vi "Lab Panel V5.27.vi"() -> ()   [LabVIEW 2013] (continued)
              w199 = T12 {"T1 Live"=20.0, "T1 Neut"=20.0, "T2 Live"=20.0, "T2 Neut"=20.0, "ID"=6.0, "ER"=10.0} ("LAB01 TEMP")
              n184 = local write "LAB deg C"(w199) -> ()
              n185 = global write "Global display 4.vi" "LAB deg C"(w199) -> ()
              n186 = local write "OFF amps"(1.5) -> ()
              n187 = local write "ON amps"(20.0) -> ()
              n188 = local write "VOLTS"(250.0) -> ()
              n189 = local write "PF"(0.5) -> ()
            }
            frame #1 {
              n190 = for {
                N: 3 -> [_]
                w245 = TRUE
                n191 = local read "Simulate"() -> (w207:bool)
                n192 = local write "Temp read loop"(0) -> ()
                n193 = case shown="True" w207 {
                  frame False {
                  }
                  frame True {
                    w247 = 20
                    n194 = local write "Ambient Volts"(2.92) -> ()
                    n195 = global write "Global display 3.vi" "Ref deg C"(w247) -> ()
                    n196 = local write "Ref deg C"(w247) -> ()
                  }
                }
                n197 = call "sub vi - GET ALL TEMP v7.vi"("LA01-EN"=w245, "simulate"=w207, "LA02-EN"=w245, "LA03-EN"=w245, "LA04-EN"=w245, "LA05-EN"=w245, "Gen Cal Value"=1) -> ("ID"=w206:T24, "LA01 TEMP"=w243:T25, "LA02 TEMP"=w236:T25, "LA03 TEMP"=w229:T25, "LA04 TEMP"=w222:T25, "LA05 TEMP"=w215:T25)  [unwired: 1 in, 2 out]
                n198 = local write "LAB05 TEMP"(w215) -> ()
                n199 = local write "LAB04 TEMP"(w222) -> ()
                n200 = Unbundle(w229) -> ("T1"=w226:dbl, "T2"=w225:dbl, "T3"=w224:dbl, "T4"=w223:dbl)  [unwired: 2 out]
                n201 = Unbundle(w243) -> ("T1"=w241:dbl, "T2"=w240:dbl, "T3"=w239:dbl, "T4"=w238:dbl)  [unwired: 2 out]
                n202 = Unbundle(w236) -> ("T1"=w233:dbl, "T2"=w232:dbl, "T3"=w231:dbl, "T4"=w230:dbl)  [unwired: 2 out]
                n203 = Unbundle(w222) -> ("T1"=w220:dbl, "T2"=w219:dbl, "T3"=w218:dbl, "T4"=w217:dbl)  [unwired: 2 out]
                n204 = Unbundle(w215) -> ("T1"=w213:dbl, "T2"=w212:dbl, "T3"=w211:dbl, "T4"=w210:dbl)  [unwired: 2 out]
                n205 = local write "LAB01 TEMP"(w243) -> ()
                n206 = local write "LAB02 TEMP"(w236) -> ()
                n207 = local write "LAB03 TEMP"(w229) -> ()
                n208 = Unbundle(w206) -> ("id1"=→"LAB01-TP":bool, "id2"=→"LAB02-TP":bool, "id3"=→"LAB03-TP":bool, "id4"=→"LAB04-TP":bool, "id5"=→"LAB05-TP":bool)
                n209 = local read "TEMP LA05"() -> (w214:T9)
                n210 = local read "TEMP LA04"() -> (w221:T9)
                n211 = local read "TEMP LA02"() -> (w235:T9)
                n212 = local read "TEMP LA03"() -> (w228:T9)
                n213 = local read "TEMP LA01"() -> (w242:T9)
                n214 = Bundle(cluster=w228, "TL-1"=w226, "TN-1"=w225, "TL-2"=w224, "TN-2"=w223) -> (w227:T9)  [unwired: 4 in]
                n215 = Bundle(cluster=w242, "TL-1"=w241, "TN-1"=w240, "TL-2"=w239, "TN-2"=w238) -> (w237:T9)  [unwired: 4 in]
                n216 = Bundle(cluster=w235, "TL-1"=w233, "TN-1"=w232, "TL-2"=w231, "TN-2"=w230) -> (w234:T9)  [unwired: 4 in]
                n217 = Bundle(cluster=w221, "TL-1"=w220, "TN-1"=w219, "TL-2"=w218, "TN-2"=w217) -> (w216:T9)  [unwired: 4 in]
                n218 = Bundle(cluster=w214, "TL-1"=w213, "TN-1"=w212, "TL-2"=w211, "TN-2"=w210) -> (w209:T9)  [unwired: 4 in]
                n219 = local write "TEMP LA03"(w227) -> ()
                n220 = local write "TEMP LA01"(w237) -> ()
                n221 = local write "TEMP LA02"(w234) -> ()
                n222 = local write "TEMP LA05"(w209) -> ()
                n223 = local write "TEMP LA04"(w216) -> ()
              }
            }
            frame #2 {
              w256 = 0
              n224 = local read "LAB01 TEMP"() -> (w258:T12)
              n225 = local read "SIG LAB01-2"() -> (w253:T2)
              n226 = Unbundle By Name(w258) -> ("T1 Live"=w251:dbl, "T1 Neut"=w250:dbl, "T2 Live"=w249:dbl, "T2 Neut"=w248:dbl)  [unwired: 2 out]
              n227 = local read "SIG LAB01-1"() -> (w255:T2)
              n228 = local read "TEMP LA01"() -> (w259:T9)
              n229 = Bundle By Name(cluster=w259, "TL-1"=w251, "TN-1"=w250, "TL-2"=w249, "TN-2"=w248, "TL -1COUNT"=w256, "TN-1 COUNT"=w256, "TL-2 COUNT"=w256, "TN-2 COUNT"=w256) -> (w257:T9)
              n230 = Bundle(cluster=w255, "Tmp Live"=w251, "Tmp Neut"=w250) -> (w254:T2)  [unwired: 3 in]
              n231 = Bundle(cluster=w253, "Tmp Live"=w249, "Tmp Neut"=w248) -> (w252:T2)  [unwired: 3 in]
              n232 = local write "SIG LAB01-2"(w252) -> ()
              n233 = local write "SIG LAB01-1"(w254) -> ()
              n234 = local write "TEMP LA01"(w257) -> ()
            }
            frame #3 {
              w268 = 0
              n235 = local read "LAB02 TEMP"() -> (w270:T12)
              n236 = Unbundle By Name(w270) -> ("T1 Live"=w263:dbl, "T1 Neut"=w262:dbl, "T2 Live"=w261:dbl, "T2 Neut"=w260:dbl)  [unwired: 2 out]
              n237 = local read "SIG LAB02-1"() -> (w267:T2)
              n238 = local read "SIG LAB02-2"() -> (w266:T2)
              n239 = local read "TEMP LA02"() -> (w271:T9)
              n240 = Bundle By Name(cluster=w271, "TL-1"=w263, "TN-1"=w262, "TL-2"=w261, "TN-2"=w260, "TL -1COUNT"=w268, "TN-1 COUNT"=w268, "TL-2 COUNT"=w268, "TN-2 COUNT"=w268) -> (w269:T9)
              n241 = Bundle(cluster=w266, "Tmp Live"=w261, "Tmp Neut"=w260) -> (w264:T2)  [unwired: 3 in]
              n242 = Bundle(cluster=w267, "Tmp Live"=w263, "Tmp Neut"=w262) -> (w265:T2)  [unwired: 3 in]
              n243 = local write "TEMP LA02"(w269) -> ()
              n244 = local write "SIG LAB02-1"(w265) -> ()
              n245 = local write "SIG LAB02-2"(w264) -> ()
            }
            frame #4 {
              w280 = 0
              n246 = local read "LAB03 TEMP"() -> (w282:T12)
              n247 = Unbundle By Name(w282) -> ("T1 Live"=w275:dbl, "T1 Neut"=w274:dbl, "T2 Live"=w273:dbl, "T2 Neut"=w272:dbl)  [unwired: 2 out]
              n248 = local read "SIG LAB03-1"() -> (w279:T2)
              n249 = local read "SIG LAB03-2"() -> (w278:T2)
              n250 = local read "TEMP LA03"() -> (w283:T9)
              n251 = Bundle By Name(cluster=w283, "TL-1"=w275, "TN-1"=w274, "TL-2"=w273, "TN-2"=w272, "TL -1COUNT"=w280, "TN-1 COUNT"=w280, "TL-2 COUNT"=w280, "TN-2 COUNT"=w280) -> (w281:T9)
              n252 = Bundle(cluster=w278, "Tmp Live"=w273, "Tmp Neut"=w272) -> (w276:T2)  [unwired: 3 in]
              n253 = Bundle(cluster=w279, "Tmp Live"=w275, "Tmp Neut"=w274) -> (w277:T2)  [unwired: 3 in]
              n254 = local write "TEMP LA03"(w281) -> ()
              n255 = local write "SIG LAB03-2"(w276) -> ()
              n256 = local write "SIG LAB03-1"(w277) -> ()
            }
            frame #5 {
              w292 = 0
              n257 = local read "LAB04 TEMP"() -> (w294:T12)
              n258 = Unbundle By Name(w294) -> ("T1 Live"=w287:dbl, "T1 Neut"=w286:dbl, "T2 Live"=w285:dbl, "T2 Neut"=w284:dbl)  [unwired: 2 out]
              n259 = local read "SIG LAB04-2"() -> (w290:T2)
              n260 = local read "SIG LAB04-1"() -> (w291:T2)
              n261 = local read "TEMP LA04"() -> (w295:T9)
              n262 = Bundle By Name(cluster=w295, "TL-1"=w287, "TN-1"=w286, "TL-2"=w285, "TN-2"=w284, "TL -1COUNT"=w292, "TN-1 COUNT"=w292, "TL-2 COUNT"=w292, "TN-2 COUNT"=w292) -> (w293:T9)
              n263 = Bundle(cluster=w290, "Tmp Live"=w285, "Tmp Neut"=w284) -> (w288:T2)  [unwired: 3 in]
              n264 = Bundle(cluster=w291, "Tmp Live"=w287, "Tmp Neut"=w286) -> (w289:T2)  [unwired: 3 in]
              n265 = local write "SIG LAB04-2"(w288) -> ()
              n266 = local write "TEMP LA04"(w293) -> ()
              n267 = local write "SIG LAB04-1"(w289) -> ()
            }
            frame #6 {
              w304 = 0
              n268 = local read "LAB05 TEMP"() -> (w306:T12)
              n269 = Unbundle By Name(w306) -> ("T1 Live"=w299:dbl, "T1 Neut"=w298:dbl, "T2 Live"=w297:dbl, "T2 Neut"=w296:dbl)  [unwired: 2 out]
              n270 = local read "SIG LAB05-2"() -> (w302:T2)
              n271 = local read "SIG LAB05-1"() -> (w303:T2)
              n272 = local read "TEMP LA05"() -> (w307:T9)
              n273 = Bundle By Name(cluster=w307, "TL-1"=w299, "TN-1"=w298, "TL-2"=w297, "TN-2"=w296, "TL -1COUNT"=w304, "TN-1 COUNT"=w304, "TL-2 COUNT"=w304, "TN-2 COUNT"=w304) -> (w305:T9)
              n274 = Bundle(cluster=w302, "Tmp Live"=w297, "Tmp Neut"=w296) -> (w300:T2)  [unwired: 3 in]
              n275 = Bundle(cluster=w303, "Tmp Live"=w299, "Tmp Neut"=w298) -> (w301:T2)  [unwired: 3 in]
              n276 = local write "SIG LAB05-2"(w300) -> ()
              n277 = local write "SIG LAB05-1"(w301) -> ()
              n278 = local write "TEMP LA05"(w305) -> ()
            }
          }
        }
        frame #11 {
          # "create analog task"
          n279 = local read "Simulate"() -> (w308:bool)
          n280 = case shown="False" w308 {
            frame False {
              n281 = local read "SAMPLES"() -> (w310:dbl)
              n282 = local read "RATE (Hz)"() -> (w311:dbl)
              n283 = local read "AI Task0"() -> (w314:dbl)
              n284 = local read "AI Task2"() -> (w312:dbl)
              n285 = local read "AI Task1"() -> (w313:dbl)
              n286 = call "sub vi - AI USB4704 (3)  Create Task v3.vi"("Task In 0"=w314, "Task In 1"=w313, "Task In 2"=w312, "Rate Hz"=w311, "Samples"=w310) -> ("TASK USB 0"=→"AI Task0":i32, "TASK USB 1"=→"AI Task1":i32, "TASK USB 2"=→"AI Task2":i32, "AI Task Er"=→"AI Task":bool)  [unwired: 6 in, 1 out]
            }
            frame True {
            }
          }
        }
        frame #12 {
          # "enable front panel, all settings done"
          n287 = property on="Tab Control 2" class="TabCtl (strict)"("DisabledEnum"=T16."Enabled" ("Disabled")) -> ()  [unwired: 2 in, 2 out]
          n288 = property on="Tab Control 2" class="TabCtl (strict)"("Value"=0) -> ()  [unwired: 2 in, 2 out]
        }
        frame #13 {
          n289 = property on="Tab Control 2" class="TabCtl (strict)"("Value"=0) -> ()  [unwired: 2 in, 2 out]
        }
      }
    }
    frame #2 {
      w321 = 250.0
      # "frames that only action on certain cycles, 13, 14, 15, 16, 19, 21"
      n290 = node-c288(w321) -> (w323:T18)  [unwired: 3 in]
      n291 = timed-loop {
        timing: w323 -> [_]
        timing-out: [_] -> w322
        tunnel: w321 -> [w324]
        i -> [w350]
        stop <- w325 stop-if-true
        n292 = node-c288() -> ()  [unwired: 1 in, 1 out]
        n293 = local read "Resets Done"() -> (w329:dbl)
        n294 = local read "SELECT LAB05-2"() -> (w330:T3)
        n295 = local read "SELECT LAB05-1"() -> (w331:T3)
        n296 = local read "SELECT LAB04-2"() -> (w332:T3)
        n297 = local read "SELECT LAB03-1"() -> (w335:T3)
        n298 = local read "SELECT LAB02-2"() -> (w336:T3)
        n299 = local read "SELECT LAB01-1"() -> (w339:T3)
        n300 = local read "SELECT LAB03-2"() -> (w334:T3)
        n301 = local read "SELECT LAB01-2"() -> (w338:T3)
        n302 = local read "SELECT LAB04-1"() -> (w333:T3)
        n303 = Greater?(x=w329, y=50) -> (0:w326:bool)
        n304 = local read "SELECT LAB02-1"() -> (w337:T3)
        n305 = local read "run lab03-2"() -> (w344:bool)
        n306 = local read "run lab04-1"() -> (w343:bool)
        n307 = local read "run lab05-1"() -> (w341:bool)
        n308 = local read "run lab04-2"() -> (w342:bool)
        n309 = local read "run lab05-2"() -> (w340:bool)
        n310 = local read "run lab03-1"() -> (w345:bool)
        n311 = local read "run lab02-2"() -> (w346:bool)
        n312 = local read "run lab02-1"() -> (w347:bool)
        n313 = local read "run lab01-1"() -> (w349:bool)
        n314 = local read "run lab01-2"() -> (w348:bool)
        n315 = Or(x=w326, y="stop") -> (x .or. y?=w325:bool)
        n316 = global write "Global display 1.vi" "stop disp"(w325) -> ()
        n317 = stacked-sequence {
          seq-local: [_ _ w429 _ _ _ _ _ _ _ _ _ _ _ _ _ _ _ _ _ _ _ _ _ _] -> [_ _ _ _ _ _ w2530 _ _ _ _ _ _ _ _ _ _ _ _ _ _ _ _ _ _]
          seq-local: [_ _ w428 _ _ _ _ _ _ _ _ _ _ _ _ _ _ _ _ _ _ _ _ _ _] -> [_ _ _ _ _ _ w2529 _ _ _ _ _ _ _ _ _ _ _ _ _ _ _ _ _ _]
          seq-local: [_ _ w415 _ _ _ _ _ _ _ _ _ _ _ _ _ _ _ _ _ _ _ _ _ _] -> [_ _ _ _ _ _ w2528 _ _ _ _ _ _ _ _ _ _ _ _ _ _ _ _ _ _]
          seq-local: [_ _ w414 _ _ _ _ _ _ _ _ _ _ _ _ _ _ _ _ _ _ _ _ _ _] -> [_ _ _ _ _ _ w2527 _ _ _ _ _ _ _ _ _ _ _ _ _ _ _ _ _ _]
          seq-local: [_ _ w413 _ _ _ _ _ _ _ _ _ _ _ _ _ _ _ _ _ _ _ _ _ _] -> [_ _ _ _ _ _ w2526 _ _ _ _ _ _ _ _ _ _ _ _ _ _ _ _ _ _]
          seq-local: [_ _ w412 _ _ _ _ _ _ _ _ _ _ _ _ _ _ _ _ _ _ _ _ _ _] -> [_ _ _ _ _ _ w2525 _ _ _ _ _ _ _ _ _ _ _ _ _ _ _ _ _ _]
          seq-local: [_ _ w411 _ _ _ _ _ _ _ _ _ _ _ _ _ _ _ _ _ _ _ _ _ _] -> [_ _ _ _ _ _ w2524 _ _ _ _ _ _ _ _ _ _ _ _ _ _ _ _ _ _]
          seq-local: [_ _ w410 _ _ _ _ _ _ _ _ _ _ _ _ _ _ _ _ _ _ _ _ _ _] -> [_ _ _ _ _ _ w2523 _ _ _ _ _ _ _ _ _ _ _ _ _ _ _ _ _ _]
          seq-local: [_ _ w409 _ _ _ _ _ _ _ _ _ _ _ _ _ _ _ _ _ _ _ _ _ _] -> [_ _ _ _ _ _ w2522 _ _ _ _ _ _ _ _ _ _ _ _ _ _ _ _ _ _]
          seq-local: [_ _ w408 _ _ _ _ _ _ _ _ _ _ _ _ _ _ _ _ _ _ _ _ _ _] -> [_ _ _ _ _ _ w2521 _ _ _ _ _ _ _ _ _ _ _ _ _ _ _ _ _ _]
          seq-local: [_ _ _ _ _ _ _ _ _ _ _ _ w3667 _ _ _ _ _ _ _ _ _ _ _ _] -> [_ _ _ _ _ _ _ _ _ _ _ _ _ w3725 _ _ _ _ _ _ _ _ _ _ _]
          tunnel: w349 -> [_ _ _ w445 w693 w2120 w2550 w2866 w3353 _ _ _ _ _ w4009 _ w4966 _ _ w5254 w5558 w5739 _ _ _]
          tunnel: w348 -> [_ _ _ w444 w691 w2119 w2549 w2867 w3352 _ _ _ _ _ w4008 _ w4964 _ _ w5253 w5557 w5737 _ _ _]
          tunnel: w347 -> [_ _ _ w443 w689 w2118 w2548 w2865 w3351 _ _ _ _ _ w4007 _ w4962 _ _ w5252 w5556 w5736 _ _ _]
          tunnel: w346 -> [_ _ _ w442 w687 w2117 w2547 w2864 w3350 _ _ _ _ _ w4006 _ w4960 _ _ w5251 w5555 w5735 _ _ _]
          tunnel: w345 -> [_ _ _ w441 w685 w2116 w2546 w2863 w3349 _ _ _ _ _ w4005 _ w4958 _ _ w5250 w5554 w5734 _ _ _]
          tunnel: w344 -> [_ _ _ w440 w683 w2115 w2545 w2862 w3348 _ _ _ _ _ w4004 _ w4956 _ _ w5249 w5553 w5733 _ _ _]
          tunnel: w343 -> [_ _ _ w439 w681 w2114 w2544 w2861 w3347 _ _ _ _ _ w4003 _ w4954 _ _ w5248 w5552 w5732 _ _ _]
          tunnel: w342 -> [_ _ _ w438 w679 w2113 w2543 w2860 w3346 _ _ _ _ _ w4002 _ w4952 _ _ w5247 w5551 w5731 _ _ _]
          tunnel: w341 -> [_ _ _ w437 w677 w2112 w2542 w2859 w3345 _ _ _ _ _ w4001 _ w4950 _ _ w5246 w5550 w5730 _ _ _]
          tunnel: w340 -> [_ _ _ w436 w675 w2111 w2541 w2858 w3344 _ _ _ _ _ w4000 _ w4948 _ _ w5245 w5549 w5729 _ _ _]
          tunnel: w339 -> [_ _ _ _ w692 w2110 w2540 _ _ _ _ _ _ _ _ _ w4968 _ _ _ _ _ w6195 _ _]
          tunnel: w338 -> [_ _ _ _ w690 w2109 w2539 _ _ _ _ _ _ _ _ _ w4963 _ _ _ _ _ w6194 _ _]
          tunnel: w337 -> [_ _ _ _ w688 w2108 w2538 _ _ _ _ _ _ _ _ _ w4961 _ _ _ _ _ w6193 _ _]
          tunnel: w336 -> [_ _ _ _ w686 w2107 w2537 _ _ _ _ _ _ _ _ _ w4959 _ _ _ _ _ w6192 _ _]
          tunnel: w335 -> [_ _ _ _ w684 w2106 w2536 _ _ _ _ _ _ _ _ _ w4957 _ _ _ _ _ w6191 _ _]
          tunnel: w334 -> [_ _ _ _ w682 w2105 w2535 _ _ _ _ _ _ _ _ _ w4955 _ _ _ _ _ w6190 _ _]
          tunnel: w333 -> [_ _ _ _ w680 w2104 w2534 _ _ _ _ _ _ _ _ _ w4953 _ _ _ _ _ w6189 _ _]
          tunnel: w332 -> [_ _ _ _ w678 w2103 w2533 _ _ _ _ _ _ _ _ _ w4951 _ _ _ _ _ w6188 _ _]
          tunnel: w331 -> [_ _ _ _ w676 w2102 w2532 _ _ _ _ _ _ _ _ _ w4949 _ _ _ _ _ w6187 _ _]
          tunnel: w330 -> [_ _ _ _ w674 w2101 w2531 _ _ _ _ _ _ _ _ _ w4947 _ _ _ _ _ w6186 _ _]
          tunnel: w326 -> [_ _ _ _ _ _ _ _ _ _ _ _ _ _ _ _ _ _ _ _ _ _ _ _ w6298]
          tunnel: w325 -> [_ _ _ _ _ _ _ _ _ _ _ _ _ _ _ _ _ _ _ _ _ _ _ _ w6297]
          tunnel: w324 -> [_ w365 _ _ _ _ _ _ _ _ _ _ _ _ _ _ _ _ _ _ _ _ _ _ _]
          frame #0 {
            n318 = local read "AI Task"() -> (w353:bool)
            n319 = global write "Global 1.vi" "RATE(Hz)"("RATE (Hz)") -> ()
            n320 = case shown="True" w353 {
              frame False {
              }
              frame True {
                n321 = local read "AI Task2"() -> (w361:dbl)
                n322 = local read "AI Task1"() -> (w362:dbl)
                n323 = local read "AI Task0"() -> (w363:dbl)
                n324 = call "sub vi - AI USB4704 (3) v73.vi"("Task0"=w363, "Task1"=w362, "Task2"=w361, "SAMPLES"="SAMPLES 2") -> ("data 0"=→"AI data 0" →"AI Data 0":waveform(dbl)[], "data 1"=→"AI data 1" →"AI Data 1":waveform(dbl)[], "data 2"=→"AI data 2" →"AI Data 2":waveform(dbl)[], "loop time"=→"AI loop time":dbl, "error array"=→"AI Error":errorcluster[])  [unwired: 7 in]
              }
            }
          }
          frame #1 {
            w372 = FALSE
            # "set up cycle control"
            n325 = local read "jig cycle"() -> (w376:dbl)
            n326 = local read "Amps Fail level"() -> (w370:dbl)
            n327 = local read "Simulate"() -> (w367:bool)
            n328 = Divide(x=w365, y=1000.0) -> (x/y=w364:dbl)
            n329 = Divide(x="JIG ON TIME (S)", y=w364) -> (x/y=→"on loops":dbl)
            n330 = Divide(x="JIG OFF TIME (S)", y=w364) -> (x/y=→"off loops":dbl)
            n331 = Increment(x=w376) -> (x+1=w375:dbl)
            n332 = local write "Simulate IND"(w367) -> ()
            n333 = global write "Global display 3.vi" "Amps Fail"(w370) -> ()
            n334 = local write "TEMP"(w372) -> ()
            n335 = local write "AI"(w372) -> ()
            n336 = local read "Network Directory"() -> (w369:path)
            n337 = local write "jig cycle"(w375) -> ()
            n338 = call "sub vi - check network dir v2.vi"("PATH"=w369) -> ("error"=w368:bool)  [unwired: 10 in]
            n339 = local write "network error"(w368) -> ()
            n340 = global write "Global display 3.vi" "network drive"(w368) -> ()
            n341 = event shown="[1] \"ADMIN\": Value Change" {
              selector: _ -> [_ _]
              dyn-events: _ -> [_ _]
              timeout: 10 -> [_ _]
              event Timeout {
                n342 = event-data() -> ()  [unwired: 1 in, 3 out]
              }
              event "ADMIN": Value Change {
                n343 = event-data() -> ()  [unwired: 1 in, 6 out]
                n344 = stacked-sequence {
                  seq-local: [_ w380 _] -> [_ _ w381]
                  frame #0 {
                    n345 = global write "Global 1.vi" "password"("9949") -> ()
                  }
                  frame #1 {
                    n346 = call "sub vi - password 1.vi"() -> ("RESULT"=w380:bool)  [unwired: 11 in]
                  }
                  frame #2 {
                    w383 = FALSE
                    n347 = property on="Tab Control 2" class="TabCtl (strict)"() -> ("Pages"=w387:refnum<vi>[])  [unwired: 2 in, 2 out]
                    n348 = Select(t=TRUE, s=w381, f=w383) -> (s? t:f=w382:bool)
                    n349 = Index Array(array=w387, index=8) -> (element=w385:refnum<vi>)
                    n350 = property class="Page"(reference=w385, "PageVis"=w382) -> ()  [unwired: 1 in, 2 out]
                    n351 = local write "ADMIN"(w383) -> ()
                  }
                }
              }
            }
          }
          frame #2 {
            w425 = 60.0
            # "convert temperature rise minutes to cycles"
            n352 = local read "SET LAB05-2"() -> (w389:T5)
            n353 = local read "SET LAB05-1"() -> (w391:T5)
            n354 = local read "SET LAB04-2"() -> (w393:T5)
            n355 = local read "SET LAB01-1"() -> (w407:T5)
            n356 = local read "SET LAB01-2"() -> (w405:T5)
            n357 = local read "SET LAB02-2"() -> (w401:T5)
            n358 = local read "SET LAB04-1"() -> (w395:T5)
            n359 = local read "SET LAB03-1"() -> (w399:T5)
            n360 = local read "SET LAB03-2"() -> (w397:T5)
            n361 = local read "SET LAB02-1"() -> (w403:T5)
            n362 = local read "JIG OFF TIME (S)"() -> (w430:dbl)
            n363 = local read "JIG ON TIME (S)"() -> (w431:dbl)
            n364 = Unbundle(w389) -> ("T-RISE mins"=w388:dbl)  [unwired: 4 out]
            n365 = Unbundle(w391) -> ("T-RISE mins"=w390:dbl)  [unwired: 4 out]
            n366 = Unbundle(w407) -> ("T-RISE mins"=w406:dbl)  [unwired: 4 out]
            n367 = Unbundle(w393) -> ("T-RISE mins"=w392:dbl)  [unwired: 4 out]
            n368 = Unbundle(w405) -> ("T-RISE mins"=w404:dbl)  [unwired: 4 out]
            n369 = Unbundle(w403) -> ("T-RISE mins"=w402:dbl)  [unwired: 4 out]
            n370 = Unbundle(w395) -> ("T-RISE mins"=w394:dbl)  [unwired: 4 out]
            n371 = Unbundle(w401) -> ("T-RISE mins"=w400:dbl)  [unwired: 4 out]
            n372 = Unbundle(w397) -> ("T-RISE mins"=w396:dbl)  [unwired: 4 out]
            n373 = Unbundle(w399) -> ("T-RISE mins"=w398:dbl)  [unwired: 4 out]
            n374 = Add(x=w431, y=w430) -> (x+y=w424:dbl)
            n375 = Multiply(x=w425, y=w396) -> (x*y=w420:dbl)
            n376 = Multiply(x=w425, y=w394) -> (x*y=w419:dbl)
            n377 = Multiply(x=w425, y=w392) -> (x*y=w418:dbl)
            n378 = Multiply(x=w425, y=w390) -> (x*y=w417:dbl)
            n379 = Multiply(x=w425, y=w388) -> (x*y=w416:dbl)
            n380 = Multiply(x=w425, y=w404) -> (x*y=w426:dbl)
            n381 = Multiply(x=w425, y=w398) -> (x*y=w421:dbl)
            n382 = Multiply(x=w425, y=w406) -> (x*y=w427:dbl)
            n383 = Multiply(x=w425, y=w402) -> (x*y=w423:dbl)
            n384 = Multiply(x=w425, y=w400) -> (x*y=w422:dbl)
            n385 = Divide(x=w417, y=w424) -> (x/y=w409:dbl)
            n386 = Divide(x=w418, y=w424) -> (x/y=w410:dbl)
            n387 = Divide(x=w419, y=w424) -> (x/y=w411:dbl)
            n388 = Divide(x=w416, y=w424) -> (x/y=w408:dbl)
            n389 = Divide(x=w421, y=w424) -> (x/y=w413:dbl)
            n390 = Divide(x=w427, y=w424) -> (x/y=w429:dbl)
            n391 = Divide(x=w426, y=w424) -> (x/y=w428:dbl)
            n392 = Divide(x=w423, y=w424) -> (x/y=w415:dbl)
            n393 = Divide(x=w422, y=w424) -> (x/y=w414:dbl)
            n394 = Divide(x=w420, y=w424) -> (x/y=w412:dbl)
          }
          frame #3 {
            # "control cycle loops"
            n395 = local read "JIG OFF TIME (S)"() -> (w434:dbl)
            n396 = local read "JIG ON TIME (S)"() -> (w433:dbl)
            n397 = local read "jig cycle"() -> (w447:dbl)
            n398 = local read "on loops"() -> (w449:dbl)
            n399 = local read "off loops"() -> (w448:dbl)
            n400 = Add(x=w434, y=w433) -> (x+y=w432:dbl)
            n401 = Add(x=w449, y=w448) -> (x+y=w435:dbl)
            n402 = Greater Or Equal?(x=w447, y=w435) -> (x >= y?=w446:bool)
            n403 = case shown="True" w446 {
              tunnel: w445 -> [_ w483]
              tunnel: w444 -> [_ w482]
              tunnel: w443 -> [_ w481]
              tunnel: w442 -> [_ w480]
              tunnel: w441 -> [_ w479]
              tunnel: w440 -> [_ w478]
              tunnel: w439 -> [_ w477]
              tunnel: w438 -> [_ w476]
              tunnel: w437 -> [_ w475]
              tunnel: w436 -> [_ w474]
              tunnel: w432 -> [_ w473]
              frame False {
              }
              frame True {
                # "increment cycle value and convert cycles to minutes for temp rise"
                n404 = stacked-sequence {
                  frame #0 {
                    n405 = local read "Temp read loop"() -> (w486:dbl)
                    n406 = Increment(x=w486) -> (x+1=w485:dbl)
                    n407 = local write "Temp read loop"(w485) -> ()
                  }
                  frame #1 {
                    n408 = local read "Temp read loop"() -> (w487:dbl)
                    n409 = Greater?(x=w487, y=20) -> (0:w489:bool)
                    n410 = case shown="True" w489 {
                      frame False {
                      }
                      frame True {
                        n411 = local write "Temp read loop"(1) -> ()
                      }
                    }
                  }
                }
                n412 = local read "JIG RELAY CYCLES"() -> (w472:T8)
                n413 = local read "Temp read loop"() -> (→"Tp Up":dbl)
                n414 = Unbundle By Name(w472) -> ("LAB01-1"=w470:dbl, "LAB01-2"=w468:dbl, "LAB02-1"=w466:dbl, "LAB02-2"=w464:dbl, "LAB03-1"=w462:dbl, "LAB03-2"=w460:dbl, "LAB04-1"=w458:dbl, "LAB04-2"=w456:dbl, "LAB05-1"=w454:dbl, "LAB05-2"=w452:dbl)
                n415 = stacked-sequence {
                  tunnel: w483 -> [w501 _ _ _ _ _ _ _ _ _]
                  tunnel: w482 -> [_ w518 _ _ _ _ _ _ _ _]
                  tunnel: w481 -> [_ _ w535 _ _ _ _ _ _ _]
                  tunnel: w480 -> [_ _ _ w552 _ _ _ _ _ _]
                  tunnel: w479 -> [_ _ _ _ w569 _ _ _ _ _]
                  tunnel: w478 -> [_ _ _ _ _ w586 _ _ _ _]
                  tunnel: w477 -> [_ _ _ _ _ _ w603 _ _ _]
                  tunnel: w476 -> [_ _ _ _ _ _ _ w620 _ _]
                  tunnel: w475 -> [_ _ _ _ _ _ _ _ w637 _]
                  tunnel: w474 -> [_ _ _ _ _ _ _ _ _ w654]
                  tunnel: w473 -> [w498 w515 w532 w549 w566 w583 w600 w617 w634 w651]
                  tunnel: w470 -> [w492 _ _ _ _ _ _ _ _ _]
                  tunnel: [w491 _ _ _ _ _ _ _ _ _] -> w469
                  tunnel: w468 -> [_ w509 _ _ _ _ _ _ _ _]
                  tunnel: [_ w508 _ _ _ _ _ _ _ _] -> w467
                  tunnel: w466 -> [_ _ w526 _ _ _ _ _ _ _]
                  tunnel: [_ _ w525 _ _ _ _ _ _ _] -> w465
                  tunnel: w464 -> [_ _ _ w543 _ _ _ _ _ _]
                  tunnel: [_ _ _ w542 _ _ _ _ _ _] -> w463
                  tunnel: w462 -> [_ _ _ _ w560 _ _ _ _ _]
                  tunnel: [_ _ _ _ w559 _ _ _ _ _] -> w461
                  tunnel: w460 -> [_ _ _ _ _ w577 _ _ _ _]
                  tunnel: [_ _ _ _ _ w576 _ _ _ _] -> w459
                  tunnel: w458 -> [_ _ _ _ _ _ w594 _ _ _]
                  tunnel: [_ _ _ _ _ _ w593 _ _ _] -> w457
                  tunnel: w456 -> [_ _ _ _ _ _ _ w611 _ _]
                  tunnel: [_ _ _ _ _ _ _ w610 _ _] -> w455
                  tunnel: w454 -> [_ _ _ _ _ _ _ _ w628 _]
                  tunnel: [_ _ _ _ _ _ _ _ w627 _] -> w453
                  tunnel: w452 -> [_ _ _ _ _ _ _ _ _ w645]
                  tunnel: [_ _ _ _ _ _ _ _ _ w644] -> w451
                  frame #0 {
                    n416 = local read "DISP LAB01-1"() -> (w496:T4)
                    n417 = Unbundle(w496) -> ("CYCLE"=w497:dbl)  [unwired: 2 out]
                    n418 = case shown="True" w501 {
                      tunnel: w497 -> [w503 w507]
                      tunnel: [w503 w506] -> w495
                      tunnel: w492 -> [w502 w505]
                      tunnel: [w502 w504] -> w491
                      frame False {
                      }
                      frame True {
                        n419 = Increment(x=w505) -> (x+1=w504:dbl)
                        n420 = Increment(x=w507) -> (x+1=w506:dbl)
                      }
                    }
                    n421 = Multiply(x=w495, y=w498) -> (x*y=w499:dbl)
                    n422 = Divide(x=w499, y=60.0) -> (x/y=w494:dbl)
                    n423 = Bundle(cluster=w496, "CYCLE"=w495, "MINS"=w494) -> (w493:T4)  [unwired: 1 in]
                    n424 = local write "DISP LAB01-1"(w493) -> ()
                  }
                  frame #1 {
                    n425 = local read "DISP LAB01-2"() -> (w513:T4)
                    n426 = Unbundle(w513) -> ("CYCLE"=w514:dbl)  [unwired: 2 out]
                    n427 = case shown="True" w518 {
                      tunnel: w514 -> [w520 w524]
                      tunnel: [w520 w523] -> w511
                      tunnel: w509 -> [w519 w522]
                      tunnel: [w519 w521] -> w508
                      frame False {
                      }
                      frame True {
                        n428 = Increment(x=w522) -> (x+1=w521:dbl)
                        n429 = Increment(x=w524) -> (x+1=w523:dbl)
                      }
                    }
                    n430 = Multiply(x=w511, y=w515) -> (x*y=w516:dbl)
                    n431 = Divide(x=w516, y=60.0) -> (x/y=w510:dbl)
                    n432 = Bundle(cluster=w513, "CYCLE"=w511, "MINS"=w510) -> (w512:T4)  [unwired: 1 in]
                    n433 = local write "DISP LAB01-2"(w512) -> ()
                  }
                  frame #2 {
                    n434 = local read "DISP LAB02-1"() -> (w530:T4)
                    n435 = Unbundle(w530) -> ("CYCLE"=w531:dbl)  [unwired: 2 out]
                    n436 = case shown="True" w535 {
                      tunnel: [w537 w541] -> w528
                      tunnel: w531 -> [w537 w540]
                      tunnel: w526 -> [w536 w539]
                      tunnel: [w536 w538] -> w525
                      frame False {
                      }
                      frame True {
                        n437 = Increment(x=w539) -> (x+1=w538:dbl)
                        n438 = Increment(x=w540) -> (x+1=w541:dbl)
                      }
                    }
                    n439 = Multiply(x=w528, y=w532) -> (x*y=w533:dbl)
                    n440 = Divide(x=w533, y=60.0) -> (x/y=w527:dbl)
                    n441 = Bundle(cluster=w530, "CYCLE"=w528, "MINS"=w527) -> (w529:T4)  [unwired: 1 in]
                    n442 = local write "DISP LAB02-1"(w529) -> ()
                  }
                  frame #3 {
                    n443 = local read "DISP LAB02-2"() -> (w547:T4)
                    n444 = Unbundle(w547) -> ("CYCLE"=w548:dbl)  [unwired: 2 out]
                    n445 = case shown="True" w552 {
                      tunnel: [w554 w558] -> w546
                      tunnel: w548 -> [w554 w557]
                      tunnel: w543 -> [w553 w556]
                      tunnel: [w553 w555] -> w542
                      frame False {
                      }
                      frame True {
                        n446 = Increment(x=w556) -> (x+1=w555:dbl)
                        n447 = Increment(x=w557) -> (x+1=w558:dbl)
                      }
                    }
                    n448 = Multiply(x=w546, y=w549) -> (x*y=w550:dbl)
                    n449 = Divide(x=w550, y=60.0) -> (x/y=w545:dbl)
                    n450 = Bundle(cluster=w547, "CYCLE"=w546, "MINS"=w545) -> (w544:T4)  [unwired: 1 in]
                    n451 = local write "DISP LAB02-2"(w544) -> ()
                  }
                  frame #4 {
                    n452 = local read "DISP LAB03-1"() -> (w564:T4)
                    n453 = Unbundle(w564) -> ("CYCLE"=w565:dbl)  [unwired: 2 out]
                    n454 = case shown="True" w569 {
                      tunnel: [w571 w575] -> w561
                      tunnel: w565 -> [w571 w574]
                      tunnel: w560 -> [w570 w573]
                      tunnel: [w570 w572] -> w559
                      frame False {
                      }
                      frame True {
                        n455 = Increment(x=w573) -> (x+1=w572:dbl)
                        n456 = Increment(x=w574) -> (x+1=w575:dbl)
                      }
                    }
                    n457 = Multiply(x=w561, y=w566) -> (x*y=w567:dbl)
                    n458 = Divide(x=w567, y=60.0) -> (x/y=w562:dbl)
                    n459 = Bundle(cluster=w564, "CYCLE"=w561, "MINS"=w562) -> (w563:T4)  [unwired: 1 in]
                    n460 = local write "DISP LAB03-1"(w563) -> ()
                  }
                  frame #5 {
                    n461 = local read "DISP LAB03-2"() -> (w581:T4)
                    n462 = Unbundle(w581) -> ("CYCLE"=w582:dbl)  [unwired: 2 out]
                    n463 = case shown="True" w586 {
                      tunnel: [w588 w592] -> w580
                      tunnel: w582 -> [w588 w591]
                      tunnel: w577 -> [w587 w590]
                      tunnel: [w587 w589] -> w576
                      frame False {
                      }
                      frame True {
                        n464 = Increment(x=w590) -> (x+1=w589:dbl)
                        n465 = Increment(x=w591) -> (x+1=w592:dbl)
                      }
                    }
                    n466 = Multiply(x=w580, y=w583) -> (x*y=w584:dbl)
                    n467 = Divide(x=w584, y=60.0) -> (x/y=w579:dbl)
                    n468 = Bundle(cluster=w581, "CYCLE"=w580, "MINS"=w579) -> (w578:T4)  [unwired: 1 in]
                    n469 = local write "DISP LAB03-2"(w578) -> ()
                  }
                  frame #6 {
                    n470 = local read "DISP LAB04-1"() -> (w598:T4)
                    n471 = Unbundle(w598) -> ("CYCLE"=w599:dbl)  [unwired: 2 out]
                    n472 = case shown="True" w603 {
                      tunnel: [w605 w609] -> w596
                      tunnel: w599 -> [w605 w608]
                      tunnel: w594 -> [w604 w607]
                      tunnel: [w604 w606] -> w593
                      frame False {
                      }
                      frame True {
                        n473 = Increment(x=w607) -> (x+1=w606:dbl)
                        n474 = Increment(x=w608) -> (x+1=w609:dbl)
                      }
                    }
                    n475 = Multiply(x=w596, y=w600) -> (x*y=w601:dbl)
                    n476 = Divide(x=w601, y=60.0) -> (x/y=w595:dbl)
                    n477 = Bundle(cluster=w598, "CYCLE"=w596, "MINS"=w595) -> (w597:T4)  [unwired: 1 in]
                    n478 = local write "DISP LAB04-1"(w597) -> ()
                  }
                  frame #7 {
                    n479 = local read "DISP LAB04-2"() -> (w615:T4)
                    n480 = Unbundle(w615) -> ("CYCLE"=w616:dbl)  [unwired: 2 out]
                    n481 = case shown="True" w620 {
                      tunnel: [w622 w626] -> w613
                      tunnel: w616 -> [w622 w625]
                      tunnel: w611 -> [w621 w624]
                      tunnel: [w621 w623] -> w610
                      frame False {
                      }
                      frame True {
                        n482 = Increment(x=w624) -> (x+1=w623:dbl)
                        n483 = Increment(x=w625) -> (x+1=w626:dbl)
                      }
                    }
                    n484 = Multiply(x=w613, y=w617) -> (x*y=w619:dbl)
                    n485 = Divide(x=w619, y=60.0) -> (x/y=w612:dbl)
                    n486 = Bundle(cluster=w615, "CYCLE"=w613, "MINS"=w612) -> (w614:T4)  [unwired: 1 in]
                    n487 = local write "DISP LAB04-2"(w614) -> ()
                  }
                  frame #8 {
                    n488 = local read "DISP LAB05-1"() -> (w632:T4)
                    n489 = Unbundle(w632) -> ("CYCLE"=w633:dbl)  [unwired: 2 out]
                    n490 = case shown="True" w637 {
                      tunnel: [w639 w643] -> w630
                      tunnel: w633 -> [w639 w642]
                      tunnel: w628 -> [w638 w641]
                      tunnel: [w638 w640] -> w627
                      frame False {
                      }
                      frame True {
                        n491 = Increment(x=w641) -> (x+1=w640:dbl)
                        n492 = Increment(x=w642) -> (x+1=w643:dbl)
                      }
                    }
                    n493 = Multiply(x=w630, y=w634) -> (x*y=w635:dbl)
                    n494 = Divide(x=w635, y=60.0) -> (x/y=w629:dbl)
                    n495 = Bundle(cluster=w632, "CYCLE"=w630, "MINS"=w629) -> (w631:T4)  [unwired: 1 in]
                    n496 = local write "DISP LAB05-1"(w631) -> ()
                  }
                  frame #9 {
                    n497 = local read "DISP LAB05-2"() -> (w650:T4)
                    n498 = Unbundle(w650) -> ("CYCLE"=w649:dbl)  [unwired: 2 out]
                    n499 = case shown="True" w654 {
                      tunnel: [w656 w660] -> w648
                      tunnel: w649 -> [w656 w659]
                      tunnel: w645 -> [w655 w658]
                      tunnel: [w655 w657] -> w644
                      frame False {
                      }
                      frame True {
                        n500 = Increment(x=w658) -> (x+1=w657:dbl)
                        n501 = Increment(x=w659) -> (x+1=w660:dbl)
                      }
                    }
                    n502 = Multiply(x=w648, y=w651) -> (x*y=w652:dbl)
                    n503 = Divide(x=w652, y=60.0) -> (x/y=w647:dbl)
                    n504 = Bundle(cluster=w650, "CYCLE"=w648, "MINS"=w647) -> (w646:T4)  [unwired: 1 in]
                    n505 = local write "DISP LAB05-2"(w646) -> ()
                  }
                }
                n506 = local write "jig cycle"(0) -> ()
                n507 = Bundle By Name(cluster=w472, "LAB01-1"=w469, "LAB01-2"=w467, "LAB02-1"=w465, "LAB02-2"=w463, "LAB03-1"=w461, "LAB03-2"=w459, "LAB04-1"=w457, "LAB04-2"=w455, "LAB05-1"=w453, "LAB05-2"=w451) -> (w471:T8)
                n508 = local write "JIG RELAY CYCLES"(w471) -> ()
              }
            }
          }
          frame #4 {
            # "START & STOP test RUN switch change, start test if true and stop test if false"
            n509 = Get Date/Time In Seconds() -> (seconds since 1Jan1904=w672:timestamp)
            n510 = local read "C drive data root dir"() -> (w665:path)
            n511 = Format Date/Time String(time format string (%c)="%b\\%a%d", seconds (now)=w672) -> (date/time string=w696:string)  [unwired: 1 in]
            n512 = Format Date/Time String(time format string (%c)="%H%M", seconds (now)=w672) -> (date/time string=w694:string)  [unwired: 1 in]
            n513 = Format Date/Time String(time format string (%c)="LabPanel%Y", seconds (now)=w672) -> (date/time string=w671:string)  [unwired: 1 in]
            n514 = Path To String(path=w665) -> (string=w668:string)
            n515 = global write "Global 1.vi" "C drive root path"(w665) -> ()
            n516 = local read "Ref deg C"() -> (w661:dbl)
            n517 = Concatenate Strings(w668, "\\") -> (w666:string)
            n518 = event shown="[1] \"RUN LAB01-1\": Value Change" {
              selector: _ -> [_ _ _ _ _ _ _ _ _ _ _]
              dyn-events: _ -> [_ _ _ _ _ _ _ _ _ _ _]
              timeout: 10 -> [_ _ _ _ _ _ _ _ _ _ _]
              tunnel: w666 -> [_ w709 w849 w990 w1130 w1270 w1410 w1550 w1690 w1830 w1971]
              tunnel: w696 -> [_ w708 w848 w989 w1129 w1269 w1409 w1549 w1689 w1829 w1970]
              tunnel: w694 -> [_ w706 w847 w988 w1128 w1268 w1408 w1548 w1688 w1828 w1969]
              tunnel: w692 -> [_ w707 _ _ _ _ _ _ _ _ _]
              tunnel: w693 -> [_ _ _ _ _ _ _ _ _ _ _]
              tunnel: w691 -> [_ _ _ _ _ _ _ _ _ _ _]
              tunnel: w690 -> [_ _ w846 _ _ _ _ _ _ _ _]
              tunnel: w689 -> [_ _ _ _ _ _ _ _ _ _ _]
              tunnel: w688 -> [_ _ _ w987 _ _ _ _ _ _ _]
              tunnel: w687 -> [_ _ _ _ _ _ _ _ _ _ _]
              tunnel: w686 -> [_ _ _ _ w1127 _ _ _ _ _ _]
              tunnel: w685 -> [_ _ _ _ _ _ _ _ _ _ _]
              tunnel: w684 -> [_ _ _ _ _ w1267 _ _ _ _ _]
              tunnel: w683 -> [_ _ _ _ _ _ _ _ _ _ _]
              tunnel: w682 -> [_ _ _ _ _ _ w1407 _ _ _ _]
              tunnel: w681 -> [_ _ _ _ _ _ _ _ _ _ _]
              tunnel: w680 -> [_ _ _ _ _ _ _ w1547 _ _ _]
              tunnel: w679 -> [_ _ _ _ _ _ _ _ _ _ _]
              tunnel: w678 -> [_ _ _ _ _ _ _ _ w1687 _ _]
              tunnel: w677 -> [_ _ _ _ _ _ _ _ _ _ _]
              tunnel: w676 -> [_ _ _ _ _ _ _ _ _ w1827 _]
              tunnel: w675 -> [_ _ _ _ _ _ _ _ _ _ _]
              tunnel: w674 -> [_ _ _ _ _ _ _ _ _ _ w1968]
              tunnel: w671 -> [_ w705 w845 w986 w1126 w1266 w1406 w1546 w1686 w1826 w1967]
              tunnel: [_ w704 w844 w985 w1125 w1265 w1405 w1545 w1685 w1825 w1966] -> w669
              tunnel: "RESET CYCLES TO ZERO?" -> [_ w703 w842 w983 w1123 w1263 w1403 w1543 w1683 w1823 w1964]
              tunnel: "YES" -> [_ w702 w841 w982 w1122 w1262 w1402 w1542 w1682 w1822 w1963]
              tunnel: "NO" -> [_ w701 w840 w981 w1121 w1261 w1401 w1541 w1681 w1821 w1962]
              tunnel: w661 -> [_ w698 w839 w979 w1120 w1260 w1400 w1540 w1680 w1820 w1960]
              event Timeout {
                n519 = event-data() -> ()  [unwired: 1 in, 3 out]
              }
              event "RUN LAB01-1": Value Change {
                n520 = event-data() -> ("NewVal"=w699:bool)  [unwired: 1 in, 5 out]
                n521 = local read "SIG LAB01-1"() -> (w700:T2)
                n522 = local write "run lab01-1"(w699) -> ()
                n523 = case shown="False" w699 {
                  tunnel: w709 -> [_ w747]
                  tunnel: w708 -> [_ w746]
                  tunnel: w707 -> [w711 w745]
                  tunnel: w706 -> [_ w744]
                  tunnel: w705 -> [_ w743]
                  tunnel: [w710 w742] -> w704
                  tunnel: w703 -> [_ w741]
                  tunnel: w702 -> [_ w740]
                  tunnel: w701 -> [_ w739]
                  tunnel: w700 -> [_ w738]
                  tunnel: w698 -> [_ w737]
                  frame False {
                    # "stop test"
                    n524 = stacked-sequence {
                      tunnel: w711 -> [_ w723 _]
                      tunnel: [_ w715 _] -> w710
                      frame #0 {
                        n525 = local read "DISP LAB01-1"() -> (w714:T4)
                        n526 = Bundle(cluster=w714, "STATUS"="STOP") -> (w712:T4)  [unwired: 2 in]
                        n527 = local write "DISP LAB01-1"(w712) -> ()
                      }
                      frame #1 {
                        n528 = local read "DISP LAB01-1"() -> (w722:T4)
                        n529 = Unbundle(w722) -> ("CYCLE"=w720:dbl, "MINS"=w721:dbl)  [unwired: 1 out]
                        n530 = case shown="\"CYCLE TEST\"" w723 {
                          tunnel: w721 -> [_ _ w730]
                          tunnel: w720 -> [w728 w729 _]
                          tunnel: [w728 w729 w730] -> w719
                          frame "CHART TEST", Default {
                          }
                          frame "CYCLE TEST" {
                          }
                          frame "T-RISE TEST" {
                          }
                        }
                        n531 = local read "TDMS LAB01-1"() -> (w727:refnum<k34>)
                        n532 = Build Array("STOPPED") -> (w724:string[])
                        n533 = Build Array(w719) -> (w718:dbl[])
                        n534 = TDMS Write(0:w727, 5:"TEST RESULT", 7:w724, 9:w718) -> (4:w716:refnum<k34>, 15:w717:errorcluster)  [unwired: 2 in, 2 out]
                        n535 = TDMS Close(8:w717, 11:w716) -> (0:w715:errorcluster)  [unwired: 1 out]
                      }
                      frame #2 {
                        n536 = stacked-sequence {
                          tunnel: "LAB01-1" -> [w733 w735]
                          frame #0 {
                            n537 = call "sub vi - defrag tdms v1.vi"("panel id"=w733) -> ("error out"=w732:errorcluster)  [unwired: 10 in]
                            n538 = local write "data file error"(w732) -> ()
                          }
                          frame #1 {
                            n539 = call "Save data file (stop) v3.vi"("panel id"=w735) -> ("network file save error"=w734:errorcluster)  [unwired: 9 in, 1 out]
                            n540 = local write "RESULT LAB01-1"(FALSE) -> ()
                            n541 = local write "data file error"(w734) -> ()
                          }
                        }
                      }
                    }
                  }
                  frame True {
                    n542 = stacked-sequence {
                      seq-local: [w749 _] -> [_ w753]
                      tunnel: w747 -> [_ w763]
                      tunnel: w746 -> [_ w762]
                      tunnel: w745 -> [_ w761]
                      tunnel: w744 -> [_ w760]
                      tunnel: w743 -> [_ w759]
                      tunnel: [_ w758] -> w742
                      tunnel: w741 -> [_ w757]
                      tunnel: w740 -> [_ w756]
                      tunnel: w739 -> [_ w755]
                      tunnel: w738 -> [w751 w754]
                      tunnel: w737 -> [_ w752]
                      frame #0 {
                        n543 = Unbundle(w751) -> ("AMPS"=w750:dbl)  [unwired: 4 out]
                        n544 = call "Check For Amps on v1.vi"("ID"="LAB01-1", "amps"=w750) -> ("amps"=w749:bool)  [unwired: 9 in]
                      }
                      frame #1 {
                        n545 = case shown="True" w753 {
                          tunnel: w763 -> [_ w776]
                          tunnel: w762 -> [_ w775]
                          tunnel: w761 -> [_ w774]
                          tunnel: w760 -> [_ w773]
                          tunnel: w759 -> [_ w772]
                          tunnel: [errorcluster {"status"=FALSE, "code"=0, "source"=""} ("error out") w771] -> w758
                          tunnel: w757 -> [_ w770]
                          tunnel: w756 -> [_ w769]
                          tunnel: w755 -> [_ w768]
                          tunnel: w754 -> [_ w767]
                          tunnel: w752 -> [_ w766]
                          frame False {
                            w764 = FALSE
                            n546 = local write "RUN LAB01-1"(w764) -> ()
                            n547 = local write "run lab01-1"(w764) -> ()
                          }
                          frame True {
                            n548 = stacked-sequence {
                              seq-local: [w777 _ _ _ _] -> [_ w798 _ _ _]
                              tunnel: w776 -> [w782 _ _ _ _]
                              tunnel: w775 -> [w778 _ _ _ _]
                              tunnel: w774 -> [w792 _ _ _ _]
                              tunnel: w773 -> [w785 _ _ _ _]
                              tunnel: w772 -> [w780 _ _ _ _]
                              tunnel: [_ w799 _ _ _] -> w771
                              tunnel: w770 -> [_ _ _ w820 _]
                              tunnel: w769 -> [_ _ _ w830 _]
                              tunnel: w768 -> [_ _ _ w829 _]
                              tunnel: w767 -> [_ _ _ _ _]
                              tunnel: w766 -> [_ _ _ _ w836]
                              frame #0 {
                                w779 = "\\"
                                n549 = case shown="\"CHART TEST\", Default" w792 {
                                tunnel: ["L01-1-CHART TEST-" "L01-1-CYCLE TEST-" "L01-1-T-RISE TEST-"] -> w788
                                frame "CHART TEST", Default {
                                }
                                frame "CYCLE TEST" {
                                }
                                frame "T-RISE TEST" {
                                }
                                }
                                n550 = local read "SET LAB01-1"() -> (w787:T5)
                                n551 = Unbundle(w787) -> ("DESCRIPTION"=w786:string)  [unwired: 4 out]
                                n552 = Concatenate Strings(w782, "\\", w780, w779, w778, w779) -> (w789:string)
                                n553 = String To Path(string=w789) -> (path=w791:path)
                                n554 = Concatenate Strings(w789, w788, w786, "-", w785, ".tdms") -> (w777:string)
                                n555 = Create Folder(path (use dialog)=w791) -> (error out=w790:errorcluster)  [unwired: 2 in, 2 out]
                                n556 = call <vilib>:"Clear Errors.vi"("error in (no error)"=w790) -> ()  [unwired: 6 in, 1 out]
                                n557 = global write "Global 1.vi" "LAB01-1 FILE"(w777) -> ()
                              }
                              frame #1 {
                                (unwired) FALSE
                                n558 = String To Path(string=w798) -> (path=w796:path)
                                n559 = TDMS Open(6:FALSE, 10:T21."create or replace" ("operation (0:open)"), 11:w796) -> (0:w799:errorcluster, 3:→"TDMS LAB01-1":refnum<k34>)  [unwired: 4 in]
                              }
                              frame #2 {
                                n560 = local read "TDMS LAB01-1"() -> (w818:refnum<k34>)
                                n561 = local read "SET LAB01-1"() -> (w807:T5)
                                n562 = Build Array("Testers Name", "Description", "Set Test Cycles", "T-Rise minutes", "T-Rise Deg C") -> (w808:string[])
                                n563 = Unbundle(w807) -> ("NAME"=w806:string, "DESCRIPTION"=w805:string, "CYCLES"=w804:dbl, "T-RISE mins"=w803:dbl, "T-RISE deg C"=w802:dbl)
                                n564 = Number To Decimal String(number=w804) -> (decimal integer string=w817:string)  [unwired: 1 in]
                                n565 = Number To Decimal String(number=w803) -> (decimal integer string=w816:string)  [unwired: 1 in]
                                n566 = Number To Decimal String(number=w802) -> (decimal integer string=w815:string)  [unwired: 1 in]
                                n567 = Build Array(w806, w805, w817, w816, w815) -> (w814:string[])
                                n568 = TDMS Set Properties(5:w814, 7:w808, 11:w818) -> ()  [unwired: 3 in, 4 out]
                              }
                              frame #3 {
                                n569 = local read "DISP LAB01-1"() -> (w828:T4)
                                n570 = Concatenate Strings("LAB01-1  ", w820) -> (w819:string)
                                n571 = Two Button Dialog(message=w819, 1:w829, 2:w830) -> (T button?=w822:bool)
                                n572 = case shown="True" w822 {
                                tunnel: w828 -> [w833 w834]
                                tunnel: [w833 w834] -> w827
                                tunnel: [w832 w835] -> w826
                                tunnel: [w831 w835] -> w825
                                frame False {
                                n573 = Unbundle(w833) -> ("CYCLE"=w832:dbl, "MINS"=w831:dbl)  [unwired: 1 out]
                                }
                                frame True {
                                w835 = 0.0
                                }
                                }
                                n574 = Bundle(cluster=w827, "CYCLE"=w826, "MINS"=w825, "STATUS"="RUN") -> (w824:T4)
                                n575 = local write "DISP LAB01-1"(w824) -> ()
                              }
                              frame #4 {
                                n576 = local read "TEMP START LAB01-1"() -> (w838:cluster{"TL":dbl, "TN":dbl})
                                n577 = Bundle(cluster=w838, "TL"=w836, "TN"=w836) -> (w837:cluster{"TL":dbl, "TN":dbl})
                                n578 = local write "TEMP START LAB01-1"(w837) -> ()
                              }
                            }
                          }
                        }
                      }
                    }
                  }
                }
              }
